vi "OM_FromLabVIEW.vi"(8 "error in (no error)":errorcluster, 11 "ObjectMap in":refnum<class "ObjectMap.lvclass">) -> (0 "error out":errorcluster, 2 "DbRow":variant, 3 "ObjectMap out":refnum<class "ObjectMap.lvclass">)   [LabVIEW 2020, in "ORM_lib.lvlib" / "ObjectMap.lvclass"]
uses:
  ObjectMap.lvclass
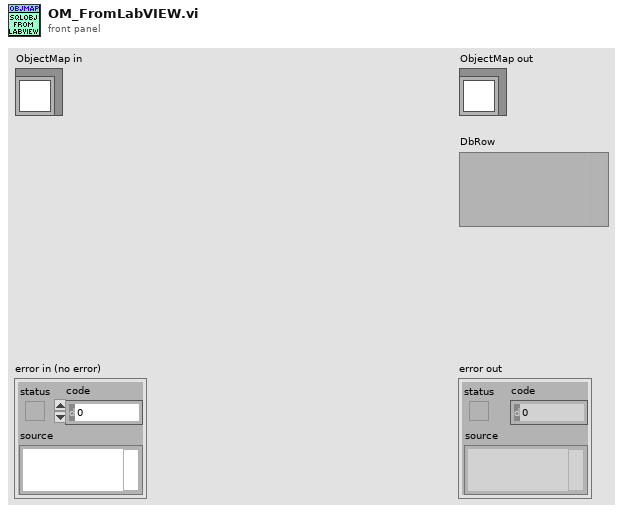
[diagram p1: front panel]
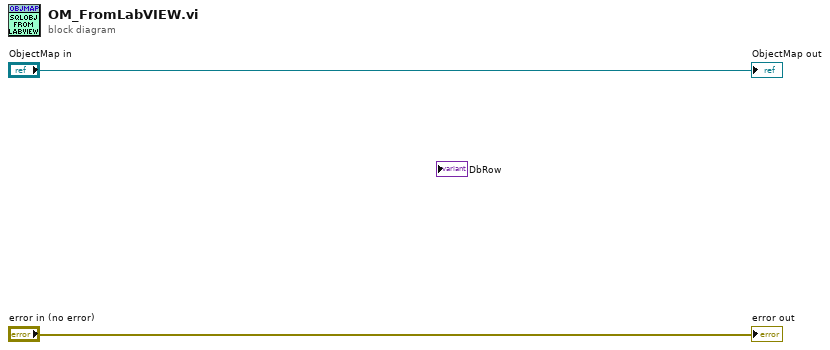
[diagram p0: block diagram]
diagram:
  "error out" <- "error in (no error)"
  "ObjectMap out" <- "ObjectMap in"
